vi "Setup.vi"(10 "Actor":refnum<class "Actor.lvclass">, 11 "Event Actor in":refnum<class "Event Actor.lvclass">) -> (3 "Event Actor out":refnum<class "Event Actor.lvclass">)   [LabVIEW 2021, in "Event Actor.lvclass"]
uses:
  Actor/Actor.lvclass
  Event Actor.lvclass
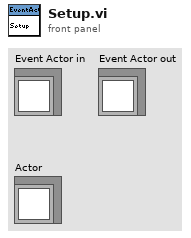
[diagram p1: front panel]
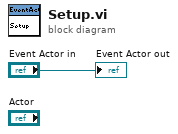
[diagram p0: block diagram]
diagram:
  "Event Actor out" <- "Event Actor in"
